vi "ProyectoBioCuinique Alpha 2.0.vi"() -> ()   [LabVIEW 2021]
uses:
  <vilib>/Utility/NIReport.llb/Report Type.ctl
  <extravilib>/ChannelInstances/Tag-dbl/Read With Abort.vi
  <extravilib>/ChannelInstances/Tag-bool/Read With Abort.vi
  <extravilib>/ChannelInstances/Tag-bool/Write With Abort.vi
  <extravilib>/ChannelInstances/Tag-dbl/Write With Abort.vi
  <vilib>/Instr/_visa.llb/VISA Configure Serial Port (Instr).vi
  <vilib>/MakerHub/LINX/Public/Utilities/Open Serial.vi
  <extravilib>/ChannelInstances/Tag-dbl/Instantiate.vi
  <extravilib>/ChannelInstances/Tag-bool/Instantiate.vi
  <extravilib>/ChannelInstances/Tag-dbl/EndpointRead.vi
  <vilib>/addons/_office/excel.llb/Excel Easy Table (str).vi
  <extravilib>/ChannelInstances/Tag-bool/EndpointRead.vi
  <extravilib>/ChannelInstances/Tag-bool/Endpoint.vi
  <extravilib>/ChannelInstances/Tag-dbl/Endpoint.vi
  <vilib>/Utility/NIReport.llb/NI_report.lvclass
  <vilib>/LabVIEW Interface for Arduino/LabVIEW Interface for Arduino.lvlib
  <vilib>/MakerHub/LINX/LMH-LINX.lvlib
  <vilib>/Utility/NIReport.llb/NI_ReportGenerationCore.lvlib
  <vilib>/addons/_office/NI_ReportGenerationToolkit.lvlib
  <vilib>/Utility/NIReport.llb/Excel/NI_Excel.lvclass
  <vilib>/MakerHub/LINX/Public/Sensors/Distance/Ultrasonic/Ultrasonic.lvlib
  <extravilib>/ChannelInstances/Tag-bool.lvlib
  <extravilib>/ChannelInstances/Tag-dbl.lvlib
panel:
  in  "template (empty)":path
  in  "Pin Bomba 1":u8
  in  "Pin Valvula 1":u8
  in  "Pin Valvula 2":u8
  out "HUMEDAD 2":dbl
  in  "VISA resource name":refnum<visa-resource-name>
  out "TEMPERATURA":dbl
  out "HUMEDAD":dbl(knob) scale=0.0..255.0
  out "Centimeters":dbl
  out "Slide":dbl(slide) scale=0.0..500.0
  out "BOMBA (11)":bool
  in  "Boolean 4":bool
  out "VALVULA (6)":bool
  in  "Boolean":bool
  out "VALVULA (5)":bool
  in  "stop":bool
  in  "VISA resource":refnum<visa-resource-name>
  # "VÁLVULA 1"
  # "BOMBA DE AGUA"
  # "VÁLVULA 2"
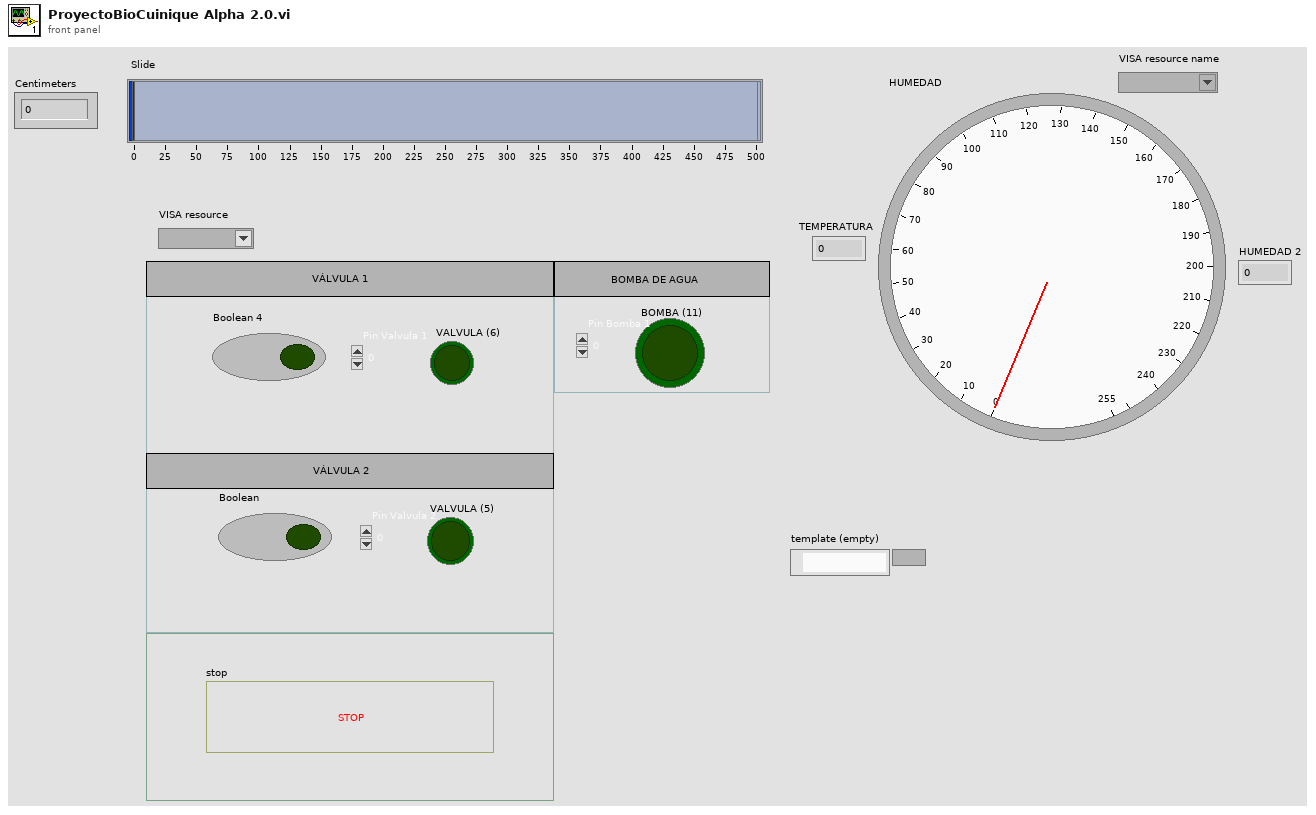
[diagram p1: front panel]
types:
  T1 = typedef "NI_ReportGenerationCore.lvlib/Report Type.ctl" = enum16{"HTML", "Word", "Excel"}
  T2 = typedef "LabVIEW Interface for Arduino.lvlib/Arduino Resource.ctl" = cluster{"VISA resource":refnum<visa-resource-name>, "Board Type":T3, "Connection Type":enum8{"USB / Serial"}, "Bytes Per Packet (15)":u8}
  T3 = typedef "LabVIEW Interface for Arduino.lvlib/Board Type.ctl" = enum16{"Uno", "Dimuelanove w/Atmega 328", "Mega 2560"}
  T4 = typedef "LMH-LINX.lvlib/LINX Ref.ctl" = cluster{"IO":T5, "Interface":T6, "LINX Device Config":T7}
  T5 = typedef "LMH-LINX.lvlib/Platform.ctl" = enum16{"Remote", "Local"}
  T6 = typedef "LMH-LINX.lvlib/Interface.ctl" = enum16{"Serial", "TCP"}
  T7 = typedef "LMH-LINX.lvlib/Device.lvlib/LINX Device Config.ctl" = cluster{"Interface":T6, "COM Port":refnum<visa-resource-name>, "TCP Configuration":T8, "Device Family":u8, "Device ID":u8, "Device Name":string, "TCP Ref":refnum<k5>, "Channels":T9}
  T8 = typedef "LMH-LINX.lvlib/Device.lvlib/TCP Config.ctl" = cluster{"IP Address":string, "Port":u16}
  T9 = typedef "LMH-LINX.lvlib/Channels.ctl" = cluster{"DI":u8[], "DO":u8[], "AI":u8[], "AO":u8[], "PWM":u8[], "QE":u8[], "UART":u8[], "I2C 2":u8[], "SPI":u8[], "CAN":u8[], "Servo":u8[], "AI Ref (V)":dbl, "AI Resolution (Bits)":u8, "AO Ref (V)":dbl, "AO Resolution (Bits)":u8}
  T10 = typedef "Tag-dbl.lvlib/))Channel.ctl" = refnum<queue>
  T11 = typedef "Tag-bool.lvlib/))Channel.ctl" = refnum<queue>
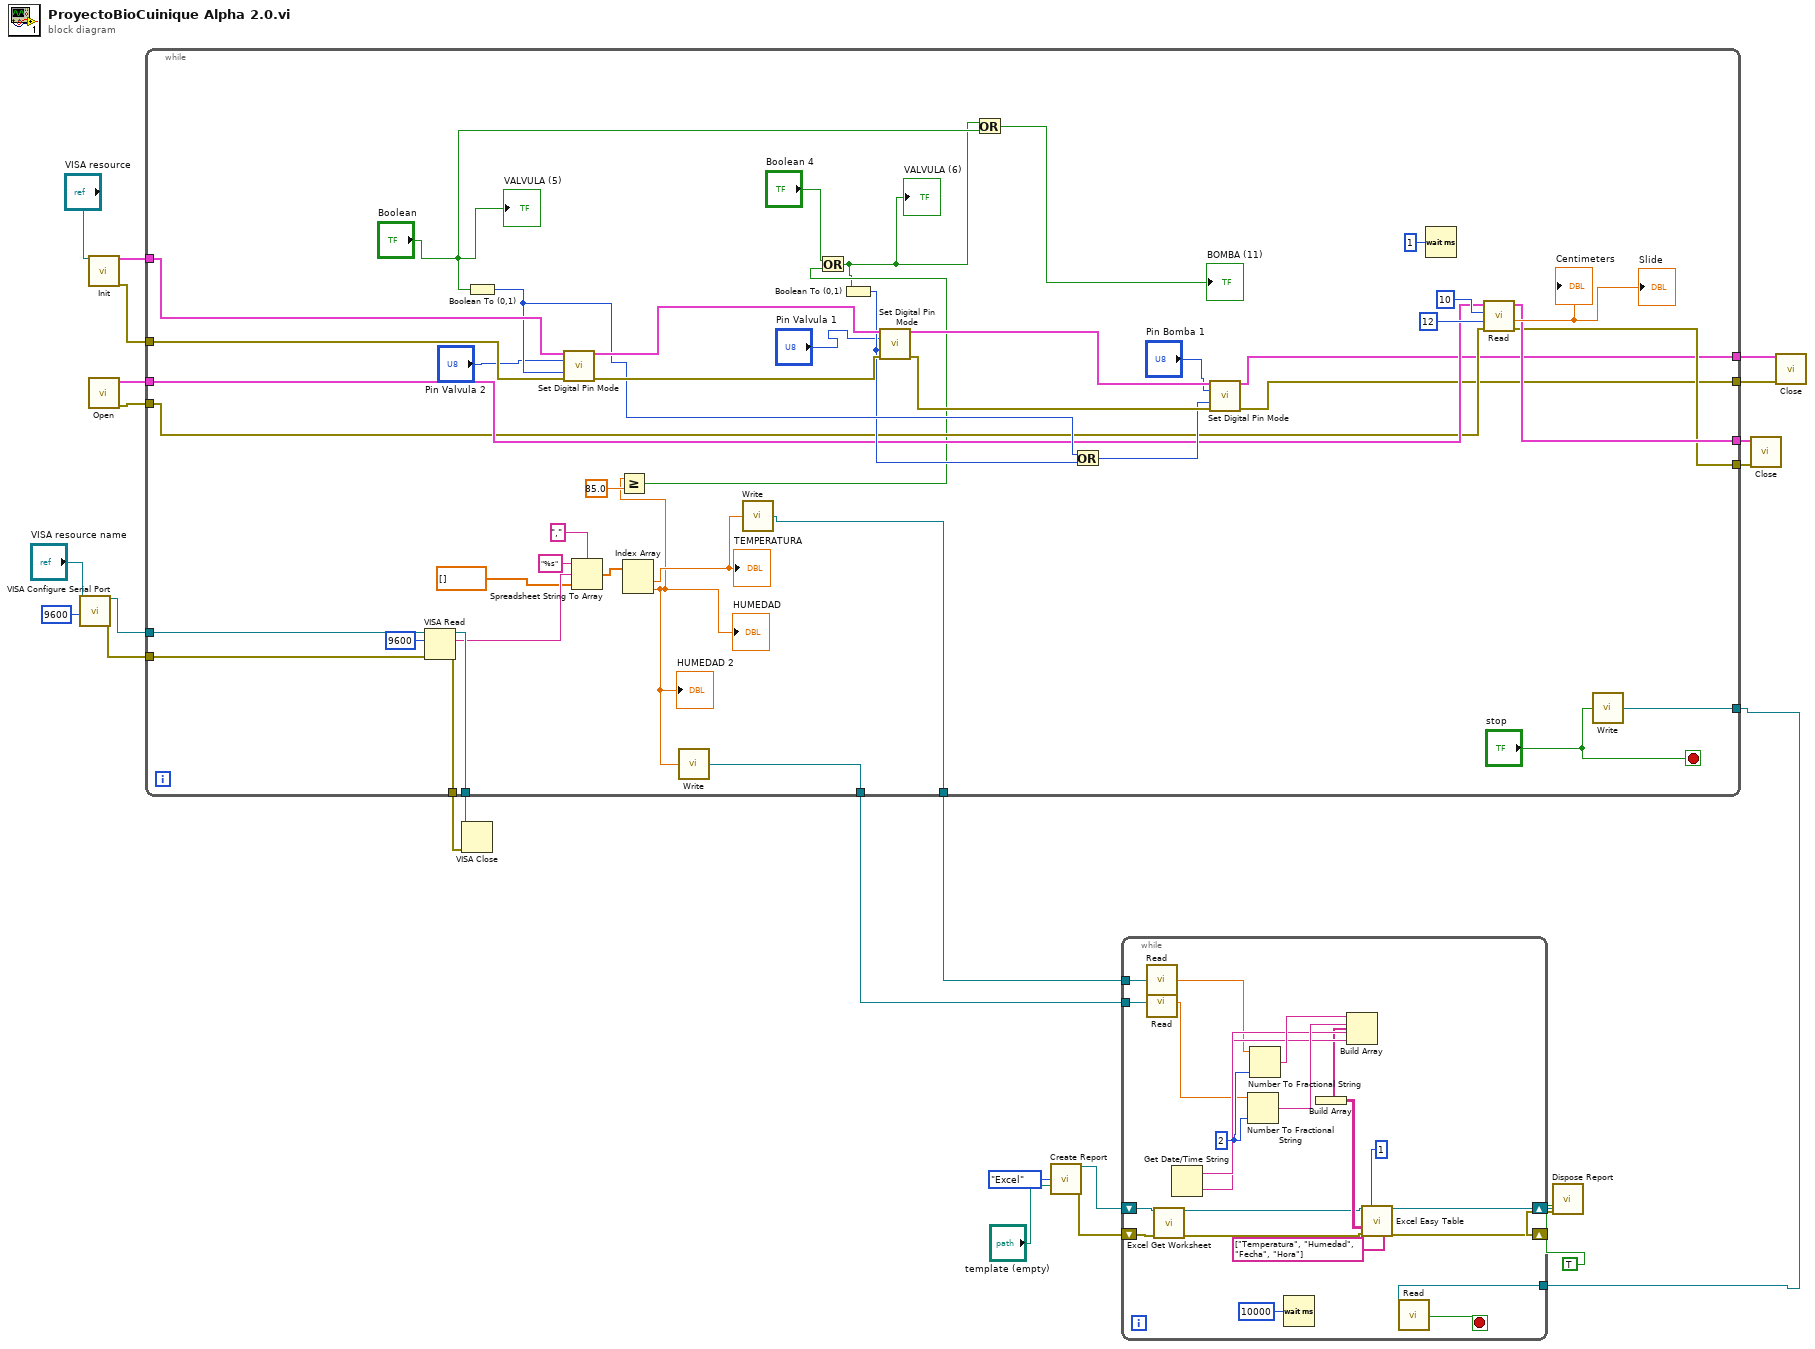
[diagram p0: block diagram]
diagram:
  n1 = call-poly "VISA Configure Serial Port"("VISA resource name"="VISA resource name", "baud rate (9600)"=u32 9600) -> ("VISA resource name out"=w16:refnum<visa-resource-name>, "error out"=w13:errorcluster)  [unwired: 12 in]
  n2 = call <vilib>:"Init.vi"("VISA resource"="VISA resource") -> ("Arduino Resource"=w24:T2, "error out"=w23:errorcluster)  [unwired: 17 in]
  n3 = call-poly <vilib>:"Open.vi"() -> ("Error Out"=w22:errorcluster, "LINX Resource"=w21:T4)  [unwired: 9 in, 1 out]
  n4 = while {
    tunnel: w24 -> [w69]
    tunnel: w23 -> [w68]
    tunnel: w22 -> [w54]
    tunnel: w21 -> [w55]
    tunnel: [w53] -> w20
    tunnel: [w52] -> w19
    tunnel: [w51] -> w18
    tunnel: [w50] -> w17
    tunnel: w16 -> [w49]
    tunnel: [w48] -> w15
    tunnel: [w47] -> w14
    tunnel: w13 -> [w46]
    tunnel: [w28] -> w3
    tunnel: [w27] -> w2
    tunnel: [w26] -> w1
    stop <- "stop" stop-if-true
    n5 = VISA Read(VISA resource name=w49, byte count=u32 9600, error in (no error)=w46) -> (VISA resource name out=w47:refnum<visa-resource-name>, read buffer=w45:string, error out=w48:errorcluster)  [unwired: 1 out]
    n6 = Boolean To (0,1)(Boolean="Boolean") -> (0, 1=w63:i16)
    n7 = call <vilib>:"Set Digital Pin Mode.vi"("Arduino Resource"=w69, "Digital I/O Pin"="Pin Valvula 2", "Pin Mode (Input)"=w63, "error in"=w68) -> ("Arduino Resource"=w67:T2, "error out"=w66:errorcluster)  [unwired: 10 in]
    n8 = Spreadsheet String To Array(delimiter (Tab)=",", format string="%s", spreadsheet string=w45, array type (2D Dbl)=dbl[] []) -> (array=w41:dbl[])
    n9 = Index Array(array=w41) -> (element #1=w40:dbl, element #2=w37:dbl)  [unwired: 2 in]
    "HUMEDAD" <- w37
    "TEMPERATURA" <- w40
    "HUMEDAD 2" <- w37
    n10 = Greater Or Equal?(x=w37, y=85.0) -> (x >= y?=w35:bool)
    n11 = call <extravilib>:"Write.vi"("element"=w37) -> ("channel"=w26:T10)  [unwired: 1 out]
    n12 = call <extravilib>:"Write.vi"("element"=w40) -> ("channel"=w27:T10)  [unwired: 1 out]
    n13 = Or(x="Boolean 4", y=w35) -> (x .or. y?=w33:bool)
    "VALVULA (6)" <- w33
    n14 = Boolean To (0,1)(Boolean=w33) -> (0, 1=w62:i16)
    n15 = call <vilib>:"Set Digital Pin Mode.vi"("Arduino Resource"=w67, "Digital I/O Pin"="Pin Valvula 1", "Pin Mode (Input)"=w62, "error in"=w66) -> ("Arduino Resource"=w64:T2, "error out"=w65:errorcluster)  [unwired: 10 in]
    n16 = Or(x=w33, y="Boolean") -> (x .or. y?=→"BOMBA (11)":bool)
    n17 = Or(x=w63, y=w62) -> (x .or. y?=w61:i16)
    n18 = call <vilib>:"Set Digital Pin Mode.vi"("Arduino Resource"=w64, "Digital I/O Pin"="Pin Bomba 1", "Pin Mode (Input)"=w61, "error in"=w65) -> ("Arduino Resource"=w51:T2, "error out"=w50:errorcluster)  [unwired: 10 in]
    n19 = Wait (ms)(milliseconds to wait=u32 1) -> ()  [unwired: 1 out]
    n20 = call <vilib>:"Read.vi"("Error In"=w54, "DO Channel"=u8 12, "DI Channel"=u8 10, "LINX Resource"=w55) -> ("Error Out"=w52:errorcluster, "Centimeters"=→"Centimeters" →"Slide":dbl, "LINX Resource"=w53:T4)  [unwired: 4 in, 1 out]
    n21 = call <extravilib>:"Write.vi"("element"="stop") -> ("channel"=w28:T11)  [unwired: 1 out]
    "VALVULA (5)" <- "Boolean"
  }
  n22 = VISA Close(VISA resource name=w14, error in (no error)=w15) -> ()  [unwired: 1 out]
  n23 = call <vilib>:"Create Report.vi"("report type"=Report_Type."Excel", "template (empty)"="template (empty)") -> ("report out"=w7:refnum<class "NI_report.lvclass">, "error out"=w8:errorcluster)  [unwired: 12 in]
  n24 = while {
    shift-right: [w79] -> w5
    shift-left: w8 -> [w84]
    shift-right: [w80] -> w6
    shift-left: w7 -> [w82]
    tunnel: w3 -> [w75]
    tunnel: w2 -> [w73]
    tunnel: w1 -> [w71]
    stop <- w74 stop-if-true
    w91 = i16 2 ("precision (6)")
    n25 = call <vilib>:"Read.vi"("channel"=w73) -> ("element"=w72:dbl)  [unwired: 1 in, 1 out]
    n26 = call <vilib>:"Read.vi"("channel"=w71) -> ("element"=w70:dbl)  [unwired: 1 in, 1 out]
    n27 = call <vilib>:"Excel Get Worksheet.vi"("report in"=w82, "error in (no error)"=w84) -> ("report out"=w81:refnum<class "NI_report.lvclass">, "error out"=w83:errorcluster)  [unwired: 12 in]
    n28 = Get Date/Time String() -> (date string=w88:string, time string=w87:string)  [unwired: 3 in]
    n29 = Number To Fractional String(number=w70, precision (6)=w91) -> (F-format string=w89:string)  [unwired: 2 in]
    n30 = Number To Fractional String(number=w72, precision (6)=w91) -> (F-format string=w90:string)  [unwired: 2 in]
    n31 = Wait (ms)(milliseconds to wait=u32 10000) -> ()  [unwired: 1 out]
    n32 = Build Array(w90, w89, w88, w87) -> (w86:string[])
    n33 = Build Array(w86) -> (w85:string[][])
    n34 = call-poly <vilib>:"Excel Easy Table.vi"("report in"=w81, "iteration"=1, "text data"=w85, "error in (no error)"=w83, "column headers"=string[] ["Temperatura", "Humedad", "Fecha", "Hora"]) -> ("report out"=w80:refnum<class "NI_report.lvclass">, "error out"=w79:errorcluster)  [unwired: 6 in, 3 out]
    n35 = call <vilib>:"Read.vi"("channel"=w75) -> ("element"=w74:bool)  [unwired: 1 in, 1 out]
  }
  n36 = call-dynamic "Dispose Report.vi"("report in"=w6, "save changes? (F)"=TRUE, "error in (no error)"=w5) -> ()  [unwired: 12 in, 1 out]
  n37 = call <vilib>:"Close.vi"("Error In"=w19, "LINX Resource"=w20) -> ()  [unwired: 9 in, 1 out]
  n38 = call <vilib>:"Close.vi"("Arduino Resource"=w18, "error in"=w17) -> ()  [unwired: 13 in, 1 out]
